vi "Main.Launcher.vi"() -> ()   [LabVIEW 2024]
uses:
  comic_manager/manager_daemon/manager_daemon.lvclass/manager_daemon.ctl
  comic_manager/manager_daemon/manager_daemon.lvclass
  <vilib>/addons/_JKI Toolkits/State Machine/_JKI_lib_State_Machine.llb/Select State(s)_err__jki_lib_state_machine.vi
  <vilib>/addons/_JKI Toolkits/State Machine/_JKI_lib_State_Machine.llb/Periodic Trigger__ogtk__JKI-SM__jki_lib_state_machine.vi
panel:
  out "manager running":bool
  in  "save indices":bool
  in  "launch crawler":bool
  in  "launch interface":bool
  in  "launch graphic UI":bool
  in  "generate indices":bool
  in  "Exit":bool
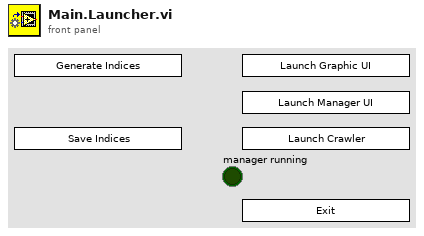
[diagram p1: front panel]
types:
  T1 = enum32{"Invalid", "Standard", "Closed", "Hidden", "Minimized", "Maximized"}
  T2 = enum32{"invalid app kind", "Development System", "Run Time System", "Student Edition", "Embedded LabVIEW", "Evaluation", "Custom"}
  T3 = cluster{"Core":cluster{"Current VI Reference":refnum<vi>, "Close Panel on Exit?":bool}, "manager_daemon":refnum<class "manager_daemon.lvclass">}
  T4 = cluster{"Current VI Reference":refnum<vi>, "Close Panel on Exit?":bool}
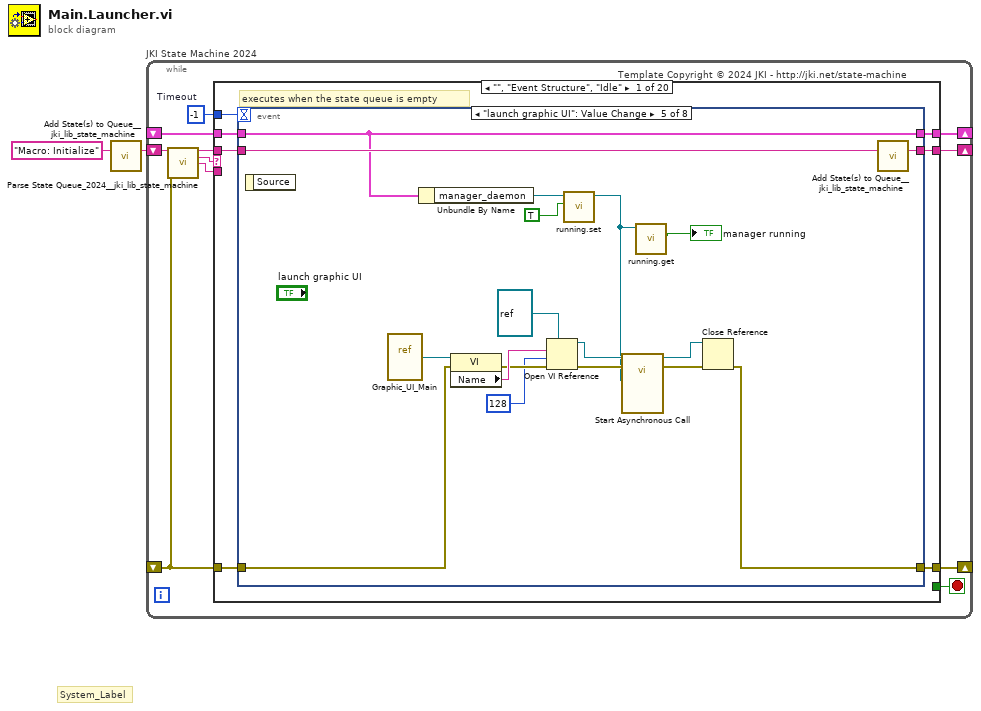
[diagram p0: block diagram]
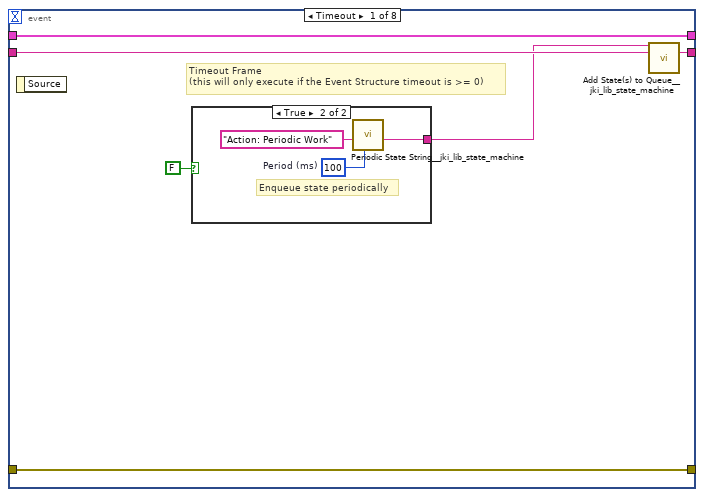
[diagram p2: hidden frame]
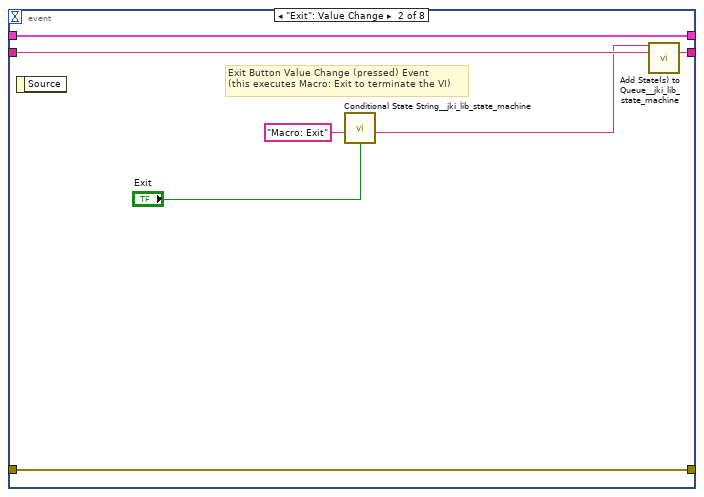
[diagram p4: hidden frame]
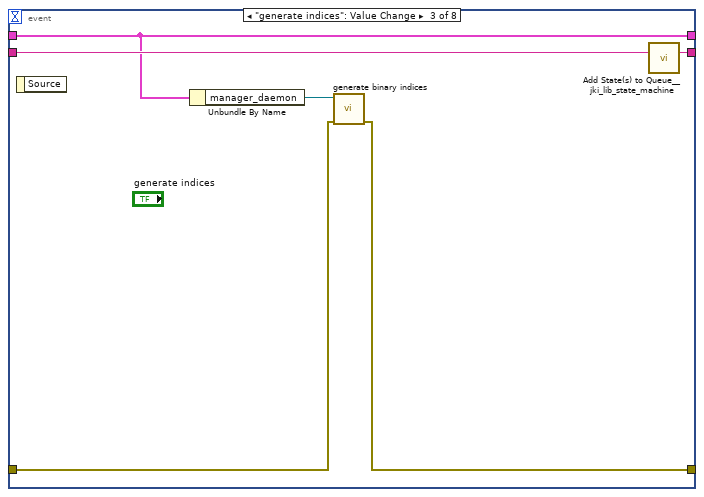
[diagram p5: hidden frame]
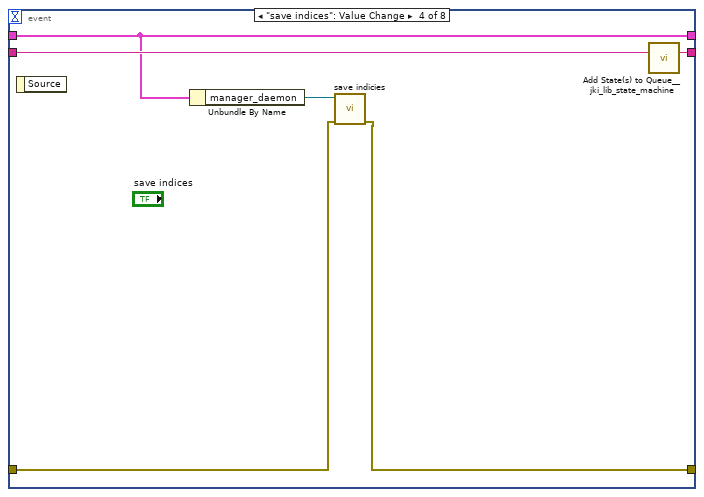
[diagram p6: hidden frame]
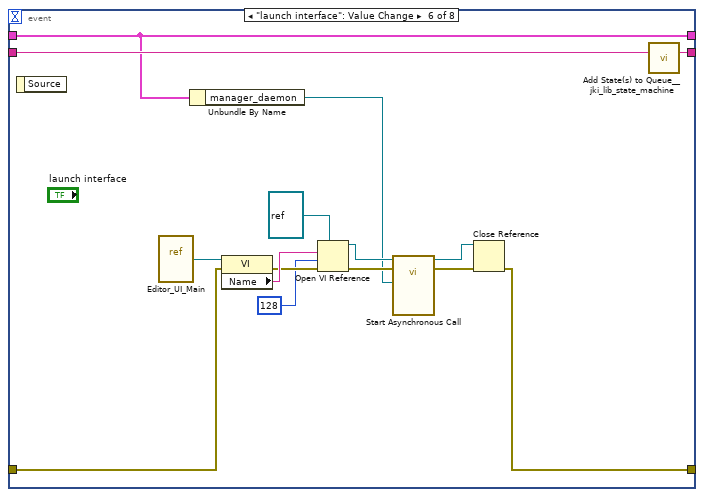
[diagram p7: hidden frame]
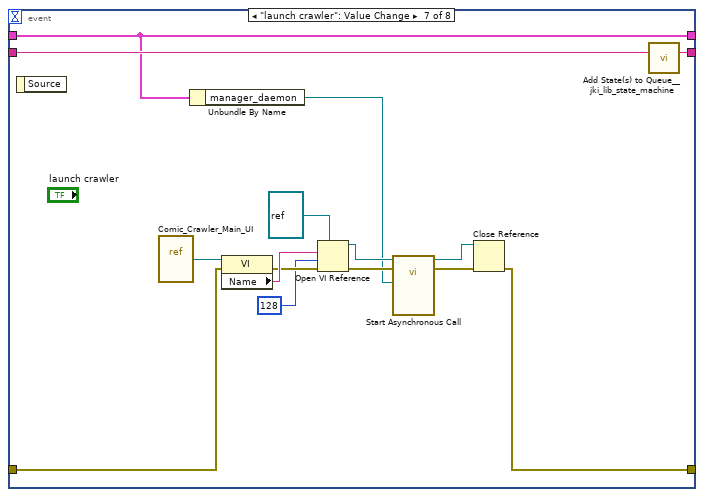
[diagram p8: hidden frame]
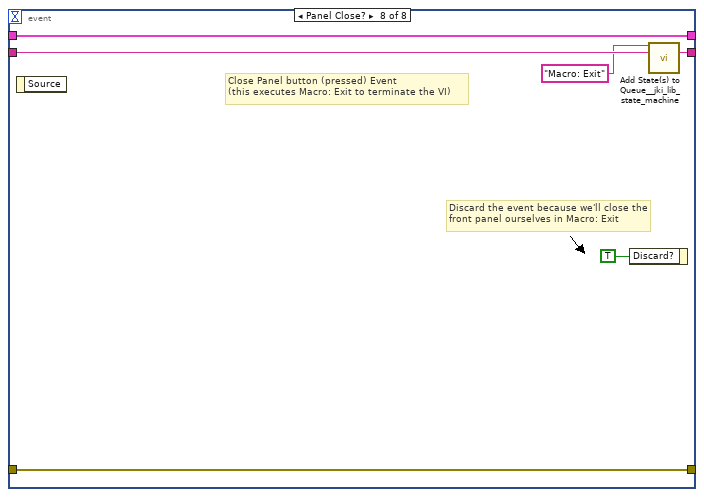
[diagram p9: hidden frame]
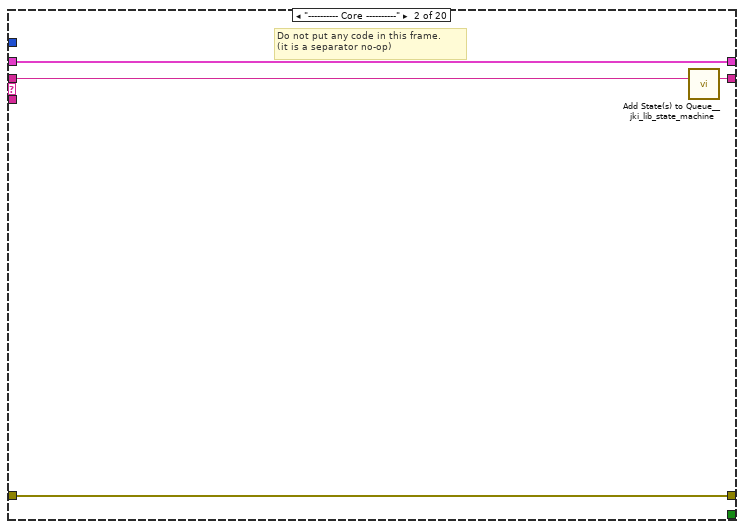
[diagram p10: hidden frame]
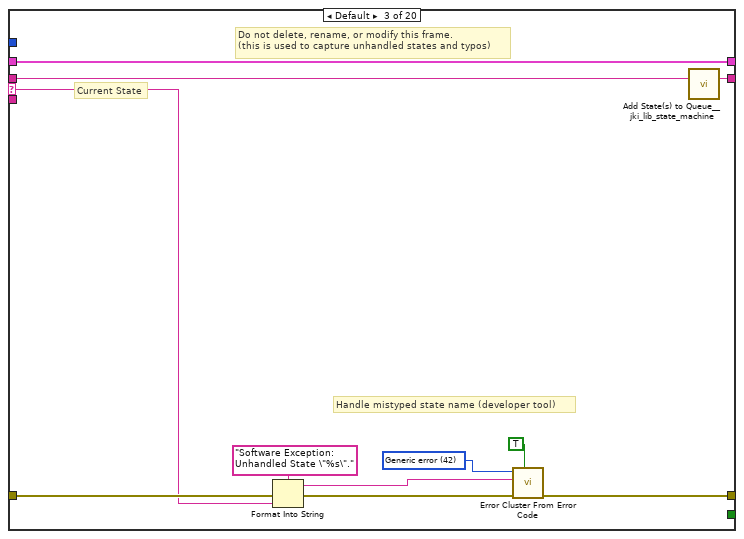
[diagram p11: hidden frame]
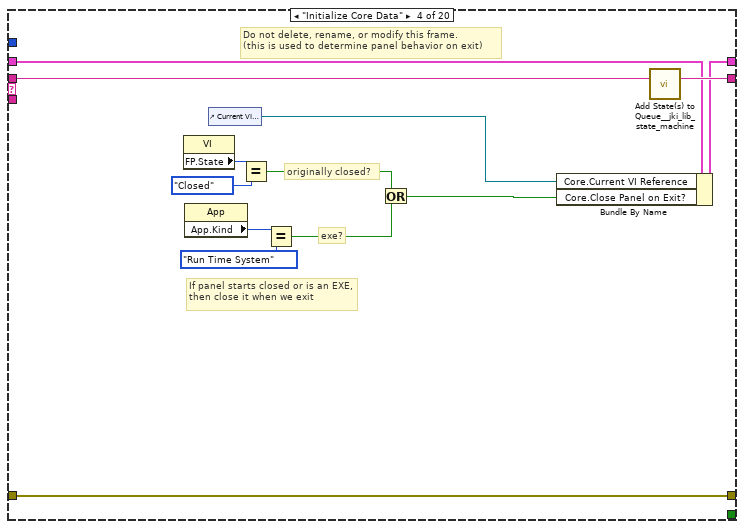
[diagram p12: hidden frame]
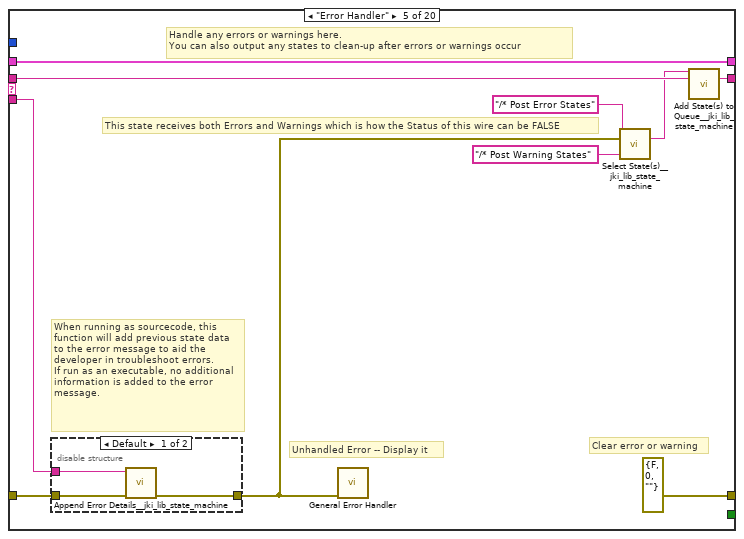
[diagram p13: hidden frame]
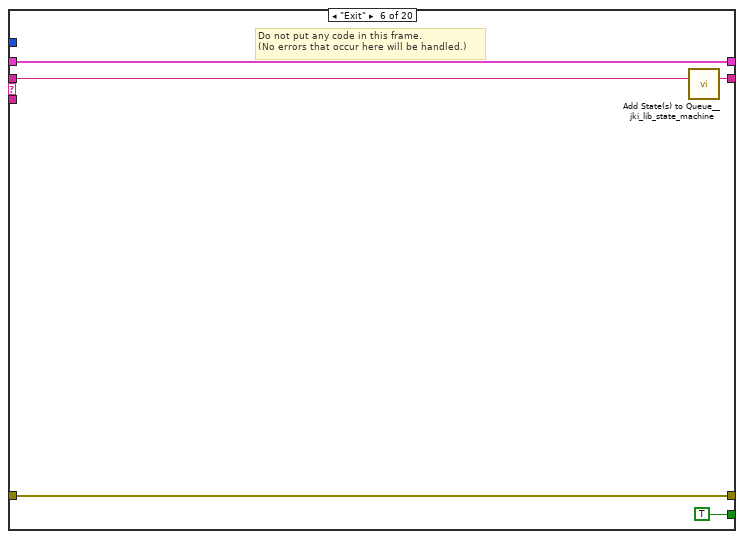
[diagram p15: hidden frame]
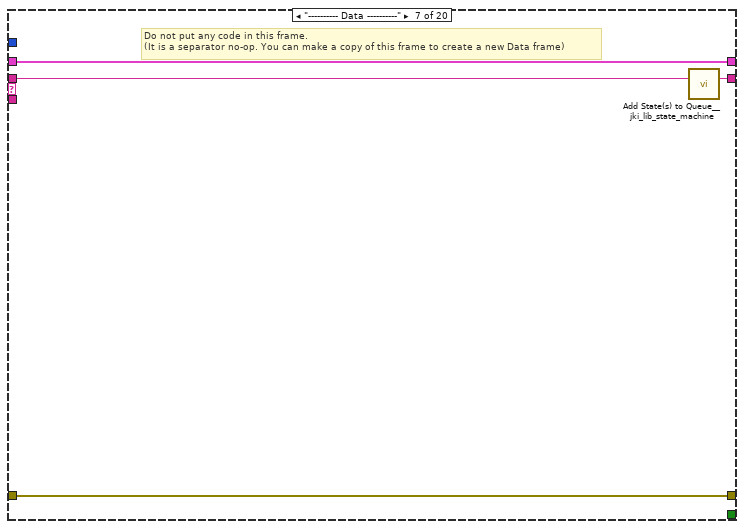
[diagram p16: hidden frame]
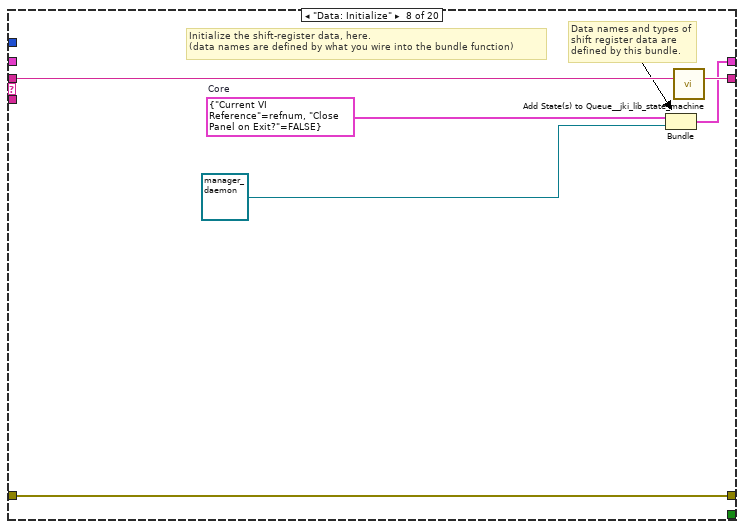
[diagram p17: hidden frame]
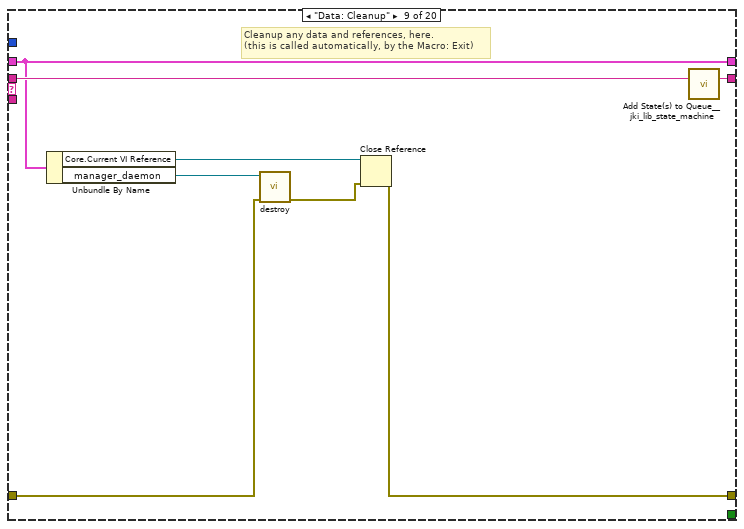
[diagram p18: hidden frame]
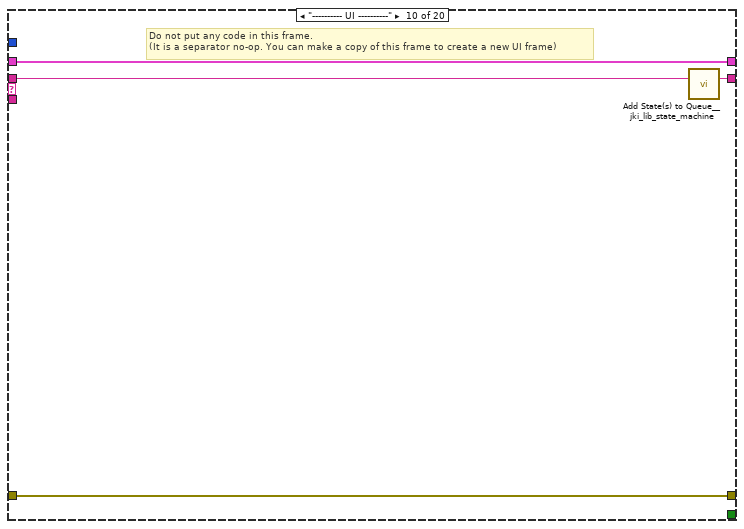
[diagram p19: hidden frame]
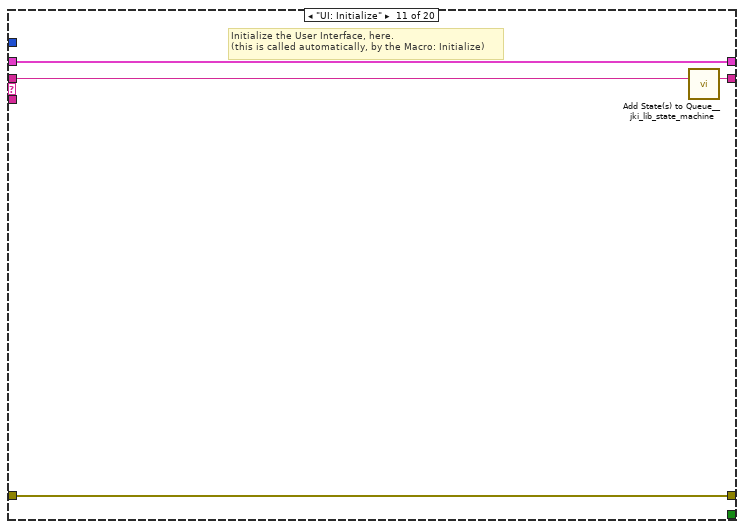
[diagram p20: hidden frame]
diagram:
  # "System_Label"
  n1 = call <vilib>:"Add State(s) to Queue__jki_lib_state_machine.vi"("State(s) in (\"\")"="Macro: Initialize") -> ("States Out"=w2:string)  [unwired: 14 in]
  n2 = while "JKI State Machine 2024" {
    shift-right: [w6] -> _
    shift-left: _ -> [w5]
    shift-right: [w9] -> _
    shift-left: _ -> [w3]
    shift-right: [w8] -> _
    shift-left: w2 -> [w10]
    stop <- w7 stop-if-true
    w4 = -1  # Timeout
    # "Template Copyright © 2024 JKI - http://jki.net/state-machine"
    n3 = call <vilib>:"Parse State Queue_2024__jki_lib_state_machine.vi"("State Queue"=w10, "Error In (no error)"=w3) -> ("Remaining States"=w12:string, "Current State"=w13:string, "Arguments"=w11:string)  [unwired: 11 in]
    n4 = case shown="\"\", \"Event Structure\", \"Idle\"" w13 {
      selector: w13 -> [_ _ w107 _ _ _ _ _ _ _ _ _ _ _ _ _ _ _ _ _]
      tunnel: w12 -> [w20 w106 w111 w130 w140 w149 w153 w159 w167 w171 w175 w179 w185 w196 w265 w270 w279 w283 w289 w300]
      tunnel: w11 -> [_ _ _ _ w135 _ _ _ _ _ _ _ w180 w190 _ _ _ _ _ _]
      tunnel: w5 -> [w18 w103 w109 w123 w137 w147 w150 _ w163 w168 w173 w177 w183 w192 w262 w267 w277 w280 w287 w292]
      tunnel: [w17 w104 w113 w127 errorcluster {"status"=FALSE, "code"=0, "source"=""} ("error out") w145 w151 w156 w164 w169 w172 w176 w181 w193 w263 w268 w271 w281 w284 w294] -> w9
      tunnel: w3 -> [w14 w104 w112 w127 w136 w145 w151 w156 w160 w169 w172 w176 w182 w194 w263 w268 w271 w281 w285 w293]
      tunnel: [w19 w105 w110 w129 w139 w148 w152 w158 w166 w170 w174 w178 w184 w195 w264 w269 w278 w282 w288 w299] -> w8
      tunnel: [_ _ _ _ _ TRUE _ _ _ _ _ _ _ _ _ _ _ _ _ _] -> w7
      tunnel: [w16 w103 w109 w128 w137 w147 w150 w157 w163 w168 w173 w177 w183 w192 w262 w267 w277 w280 w287 w290] -> w6
      tunnel: w4 -> [w15 _ _ _ _ _ _ _ _ _ _ _ _ _ _ _ _ _ _ _]
      frame "", "Event Structure", "Idle" {
        # "executes when the state queue is empty"
        n5 = event shown="[4] \"launch graphic UI\": Value Change" {
          selector: _ -> [_ _ _ _ _ _ _ _]
          dyn-events: _ -> [_ _ _ _ _ _ _ _]
          timeout: w15 -> [_ _ _ _ _ _ _ _]
          tunnel: w20 -> [w26 w36 w42 w48 w66 w81 w96 w102]
          tunnel: [w25 w35 w41 w47 w65 w80 w95 w101] -> w19
          tunnel: w18 -> [w23 w33 w40 w46 w64 w79 w94 w99]
          tunnel: [w24 w34 w37 w43 w53 w67 w82 w100] -> w17
          tunnel: w14 -> [w24 w34 w38 w44 w54 w69 w84 w100]
          tunnel: [w23 w33 w40 w46 w64 w79 w94 w99] -> w16
          event Timeout {
            # "Timeout Frame\n(this will only execute if the Event Structure timeout is >= 0)"
            n6 = event-data() -> ()  [unwired: 1 in, 1 out]
            n7 = case shown="True" FALSE {
              tunnel: [_ w29] -> w22
              frame False {
              }
              frame True {
                w27 = u32 100  # Period (ms)
                # "Enqueue state periodically"
                n8 = call <vilib>:"Periodic State String__jki_lib_state_machine.vi"("Period (ms)"=w27, "State"="Action: Periodic Work") -> ("State Out"=w29:string)  [unwired: 9 in]
              }
            }
            n9 = call <vilib>:"Add State(s) to Queue__jki_lib_state_machine.vi"("State(s) in Front (\"\")"=w22, "State(s) in (\"\")"=w26) -> ("States Out"=w25:string)  [unwired: 13 in]
          }
          event "Exit": Value Change {
            # "Exit Button Value Change (pressed) Event\n(this executes Macro: Exit to terminate the VI)"
            n10 = event-data() -> ()  [unwired: 1 in, 1 out]
            n11 = call <vilib>:"Conditional State String__jki_lib_state_machine.vi"("Do State(s)?"="Exit", "State"="Macro: Exit") -> ("State Out"=w30:string)  [unwired: 7 in]
            n12 = call <vilib>:"Add State(s) to Queue__jki_lib_state_machine.vi"("State(s) in Front (\"\")"=w30, "State(s) in (\"\")"=w36) -> ("States Out"=w35:string)  [unwired: 13 in]
          }
          event "generate indices": Value Change {
            n13 = event-data() -> ()  [unwired: 1 in, 1 out]
            n14 = Unbundle By Name(w40) -> ("manager_daemon"=w39:refnum<class "manager_daemon.lvclass">)
            n15 = call "generate binary indices.vi"("error in (no error)"=w38, "manager_daemon in"=w39) -> ("error out"=w37:errorcluster)  [unwired: 8 in, 1 out]
            n16 = call <vilib>:"Add State(s) to Queue__jki_lib_state_machine.vi"("State(s) in (\"\")"=w42) -> ("States Out"=w41:string)  [unwired: 14 in]
          }
          event "save indices": Value Change {
            n17 = event-data() -> ()  [unwired: 1 in, 1 out]
            n18 = Unbundle By Name(w46) -> ("manager_daemon"=w45:refnum<class "manager_daemon.lvclass">)
            n19 = call "save indicies.vi"("error in (no error)"=w44, "manager_daemon in"=w45) -> ("error out"=w43:errorcluster)  [unwired: 8 in, 1 out]
            n20 = call <vilib>:"Add State(s) to Queue__jki_lib_state_machine.vi"("State(s) in (\"\")"=w48) -> ("States Out"=w47:string)  [unwired: 14 in]
          }
          event "launch graphic UI": Value Change {
            n21 = event-data() -> ()  [unwired: 1 in, 1 out]
            n22 = vi-ref "Graphic_UI_Main.vi"() -> (w56:refnum<vi>)
            n23 = Unbundle By Name(w64) -> ("manager_daemon"=w51:refnum<class "manager_daemon.lvclass">)
            n24 = property class="VI"(reference=w56, error in=w54) -> (error out=w57:errorcluster, "Name"=w58:string)  [unwired: 1 out]
            n25 = Open VI Reference(type specifier VI Refnum (for type only)=refnum<vi> refnum, vi path=w58, options=128, error in (no error)=w57) -> (vi reference=w60:refnum<vi>, error out=w63:errorcluster)  [unwired: 2 in]
            n26 = call "running.set.vi"("running"=TRUE, "manager_daemon in"=w51) -> ("manager_daemon out"=w50:refnum<class "manager_daemon.lvclass">)  [unwired: 9 in]
            n27 = call-by-ref "Start Asynchronous Call"(reference=w60, error in=w63, "manager_daemon"=w50) -> (reference out=w61:refnum<vi>, error out=w62:errorcluster)  [unwired: 11 in]
            n28 = call "running.get.vi"("manager_daemon in"=w50) -> ("manager running"=→"manager running":bool)  [unwired: 9 in, 1 out]
            n29 = Close Reference(reference=w61, error in (no error)=w62) -> (error out=w53:errorcluster)
            n30 = call <vilib>:"Add State(s) to Queue__jki_lib_state_machine.vi"("State(s) in (\"\")"=w66) -> ("States Out"=w65:string)  [unwired: 14 in]
          }
          event "launch interface": Value Change {
            n31 = event-data() -> ()  [unwired: 1 in, 1 out]
            n32 = vi-ref "Editor_UI_Main.vi"() -> (w71:refnum<vi>)
            n33 = Unbundle By Name(w79) -> ("manager_daemon"=w68:refnum<class "manager_daemon.lvclass">)
            n34 = property class="VI"(reference=w71, error in=w69) -> (error out=w72:errorcluster, "Name"=w73:string)  [unwired: 1 out]
            n35 = Open VI Reference(type specifier VI Refnum (for type only)=refnum<vi> refnum, vi path=w73, options=128, error in (no error)=w72) -> (vi reference=w75:refnum<vi>, error out=w78:errorcluster)  [unwired: 2 in]
            n36 = call-by-ref "Start Asynchronous Call"(reference=w75, error in=w78, "manager_daemon"=w68) -> (reference out=w76:refnum<vi>, error out=w77:errorcluster)  [unwired: 11 in]
            n37 = Close Reference(reference=w76, error in (no error)=w77) -> (error out=w67:errorcluster)
            n38 = call <vilib>:"Add State(s) to Queue__jki_lib_state_machine.vi"("State(s) in (\"\")"=w81) -> ("States Out"=w80:string)  [unwired: 14 in]
          }
          event "launch crawler": Value Change {
            n39 = event-data() -> ()  [unwired: 1 in, 1 out]
            n40 = vi-ref "Comic_Crawler_Main_UI.vi"() -> (w86:refnum<vi>)
            n41 = Unbundle By Name(w94) -> ("manager_daemon"=w83:refnum<class "manager_daemon.lvclass">)
            n42 = property class="VI"(reference=w86, error in=w84) -> (error out=w87:errorcluster, "Name"=w88:string)  [unwired: 1 out]
            n43 = Open VI Reference(type specifier VI Refnum (for type only)=refnum<vi> refnum, vi path=w88, options=128, error in (no error)=w87) -> (vi reference=w90:refnum<vi>, error out=w93:errorcluster)  [unwired: 2 in]
            n44 = call-by-ref "Start Asynchronous Call"(reference=w90, error in=w93, "manager_daemon"=w83) -> (reference out=w91:refnum<vi>, error out=w92:errorcluster)  [unwired: 11 in]
            n45 = Close Reference(reference=w91, error in (no error)=w92) -> (error out=w82:errorcluster)
            n46 = call <vilib>:"Add State(s) to Queue__jki_lib_state_machine.vi"("State(s) in (\"\")"=w96) -> ("States Out"=w95:string)  [unwired: 14 in]
          }
          event Panel Close? {
            # "Discard the event because we'll close the front panel ourselves in Macro: Exit"
            # "Close Panel button (pressed) Event\n(this executes Macro: Exit to terminate the VI)"
            n47 = event-data() -> ()  [unwired: 1 in, 1 out]
            n48 = event-data("Discard?"=TRUE) -> ()  [unwired: 1 in, 1 out]
            n49 = call <vilib>:"Add State(s) to Queue__jki_lib_state_machine.vi"("State(s) in Front (\"\")"="Macro: Exit", "State(s) in (\"\")"=w102) -> ("States Out"=w101:string)  [unwired: 13 in]
          }
        }
      }
      frame "---------- Core ----------" {
        # "Do not put any code in this frame.\n(it is a separator no-op)"
        n50 = call <vilib>:"Add State(s) to Queue__jki_lib_state_machine.vi"("State(s) in (\"\")"=w106) -> ("States Out"=w105:string)  [unwired: 14 in]
      }
      frame Default {
        w116 = 42 items=["No error", "Argument error", "Memory is full", "Out of zone", "End of file", "File already open", "Generic file I/O error", "File not found", "File permission error", "Disk is full", "Duplicate path", "Too many files open", "System feature not enabled", "Resource file not found", "Cannot add resource", "Resource not found", "Image not found", "Image memory error", "Pen does not exist", "Config type invalid", "Config token not found", "Config parse error", "Config memory error", "Bad external code format", "Bad external code offset", "External code not present", "Null window", "Destroy window error", "Null menu", "Print aborted", "Bad print record", "Print driver error", "Windows error during printing", "Memory error during printing", "Print dialog error", "Generic print error", "Invalid device refnum", "Device not found", "Device parameter error", "Device unit error", "Cannot open device", "Device call aborted", "Generic error", "Cancelled by user", "Object ID too low", "Object ID too high", "Object not in heap", "Unknown heap", "Unknown object (invalid DefProc)", "Unknown object (DefProc not in table)", "Message out of range", "Invalid (null) method", "Unknown message", "Manager call not supported", "Bad address", "Network operation in progress", "Network operation timed out", "Connection is busy", "Network attribute not supported", "Network error", "Address in use", "System out of memory", "Connection aborted", "Connection refused", "Not connected", "Already connected", "Connection closed", "Initialization error (interapplication manager)", "Bad occurrence", "Wait on unbound occurrence handler", "Occurrence queue overflow", "Datalog type conflict", "Unused", "Unrecognized type (interapplication manager)", "Memory corrupt", "Failed to make temporary DLL", "Old CIN version", "Drag socket not found", "Failed to load drop-object", "Failed to register OLE object", "Failed to release OLE object", "Format specifier type mismatch", "Unknown format specifier", "Too few format specifiers", "Too many format specifiers", "Scan failed", "Newer CIN version", "Error converting to variant", "Runtime menu error", "Password tampered", "Variant attribute not found", "Incompatible variant data type", "Event data is not available", "Event Store is not present", "Occurrence is not found", "Event Queue is not created", "Event info is not available", "Refnum passed is NULL", "Error retrieving Class GUID", "Error retrieving CoClass GUID", "Error retrieving TypeLib GUID.", "Bad built application magic bytes.", "Specific driver is different from the specific driver associated with the Logical Name.", "There is no session opened to the class driver.", "Max Error", "MAX - Error with config objects", "MAX - Error loading configuration", "MAX - Group not supported"]
        # "Current State"
        # "Do not delete, rename, or modify this frame.\n(this is used to capture unhandled states and typos)"
        # "Handle mistyped state name (developer tool)"
        n51 = Format Into String(format string="Software Exception: Unhandled State \"%s\"." ("message"), error in=w112, w107) -> (resulting string=w115:string, error out=w114:errorcluster)  [unwired: 1 in]
        n52 = call <vilib>:"Error Cluster From Error Code.vi"("show call chain? (False)"=TRUE, "error in (no error)"=w114, "error message (\"\")"=w115, "error code (0)"=w116) -> ("error out"=w113:errorcluster)  [unwired: 5 in]
        n53 = call <vilib>:"Add State(s) to Queue__jki_lib_state_machine.vi"("State(s) in (\"\")"=w111) -> ("States Out"=w110:string)  [unwired: 14 in]
      }
      frame "Initialize Core Data" {
        # "Do not delete, rename, or modify this frame.\n(this is used to determine panel behavior on exit)"
        # "originally closed?"
        # "exe?"
        # "If panel starts closed or is an EXE, then close it when we exit"
        n54 = property class="VI"() -> ("FP.State"=w120:T1)  [unwired: 2 in, 2 out]
        n55 = property class="App"() -> ("App.Kind"=w126:T2)  [unwired: 2 in, 2 out]
        n56 = control-ref of="Current VI Reference"() -> (w121:refnum<vi>)
        n57 = Equal?(x=w120, y=T1."Closed" ("Front Panel Window:State")) -> (x = y?=w118:bool)
        n58 = Equal?(x=w126, y=T2."Run Time System" ("Application:Kind")) -> (x = y?=w124:bool)
        n59 = Or(x=w118, y=w124) -> (x .or. y?=w122:bool)
        n60 = Bundle By Name(cluster=w123, "Core.Current VI Reference"=w121, "Core.Close Panel on Exit?"=w122) -> (w128:T3)
        n61 = call <vilib>:"Add State(s) to Queue__jki_lib_state_machine.vi"("State(s) in (\"\")"=w130) -> ("States Out"=w129:string)  [unwired: 14 in]
      }
      frame "Error Handler" {
        # "When running as sourcecode, this function will add previous state data to the error message to aid the developer in troubleshoot errors.\nIf run as an executable, no additional information is added to the error message."
        # "This state receives both Errors and Warnings which is how the Status of this wire can be FALSE"
        # "Unhandled Error -- Display it"
        # "Handle any errors or warnings here.\nYou can also output any states to clean-up after errors or warnings occur"
        # "Clear error or warning"
        n62 = disable-structure shown="Default" {
          disable-tunnel: w136 -> [w143 w144]
          disable-tunnel: w135 -> [w142 _]
          disable-tunnel: [w141 w144] -> w134
          frame condition #0 (active) {
            n63 = call <vilib>:"Append Error Details__jki_lib_state_machine.vi"("error in (no error)"=w143, "Previous State and Argument(s)"=w142) -> ("error out"=w141:errorcluster)  [unwired: 9 in]
          }
          frame condition #1 {
          }
        }
        n64 = call <vilib>:"General Error Handler.vi"("error in (no error)"=w134) -> ()  [unwired: 10 in, 5 out]
        n65 = call-poly <vilib>:"Select State(s)__jki_lib_state_machine.vi"("State(s) if True (\"\")"="/* Post Error States", "Select"=w134, "State(s) if False (\"\")"="/* Post Warning States") -> ("States Out"=w132:string)  [unwired: 12 in]
        n66 = call <vilib>:"Add State(s) to Queue__jki_lib_state_machine.vi"("State(s) in Front (\"\")"=w132, "State(s) in (\"\")"=w140) -> ("States Out"=w139:string)  [unwired: 13 in]
      }
      frame "Exit" {
        # "Do not put any code in this frame.\n(No errors that occur here will be handled.)"
        n67 = call <vilib>:"Add State(s) to Queue__jki_lib_state_machine.vi"("State(s) in (\"\")"=w149) -> ("States Out"=w148:string)  [unwired: 14 in]
      }
      frame "---------- Data ----------" {
        # "Do not put any code in this frame.\n(It is a separator no-op. You can make a copy of this frame to create a new Data frame)"
        n68 = call <vilib>:"Add State(s) to Queue__jki_lib_state_machine.vi"("State(s) in (\"\")"=w153) -> ("States Out"=w152:string)  [unwired: 14 in]
      }
      frame "Data: Initialize" {
        w155 = T4 {"Current VI Reference"=refnum, "Close Panel on Exit?"=FALSE}  # Core
        # "Data names and types of shift register data are defined by this bundle."
        # "Initialize the shift-register data, here.\n(data names are defined by what you wire into the bundle function)"
        n69 = Bundle("Core"=w155, "manager_daemon"=refnum<class "manager_daemon.lvclass"> refnum) -> (w157:T3)  [unwired: 1 in]
        n70 = call <vilib>:"Add State(s) to Queue__jki_lib_state_machine.vi"("State(s) in (\"\")"=w159) -> ("States Out"=w158:string)  [unwired: 14 in]
      }
      frame "Data: Cleanup" {
        # "Cleanup any data and references, here.\n(this is called automatically, by the Macro: Exit)"
        n71 = Unbundle By Name(w163) -> ("Core.Current VI Reference"=w165:refnum<vi>, "manager_daemon"=w162:refnum<class "manager_daemon.lvclass">)
        n72 = call "destroy.vi"("error in (no error)"=w160, "manager_daemon in"=w162) -> ("error out"=w161:errorcluster)  [unwired: 8 in, 1 out]
        n73 = Close Reference(reference=w165, error in (no error)=w161) -> (error out=w164:errorcluster)
        n74 = call <vilib>:"Add State(s) to Queue__jki_lib_state_machine.vi"("State(s) in (\"\")"=w167) -> ("States Out"=w166:string)  [unwired: 14 in]
      }
      frame "---------- UI ----------" {
        # "Do not put any code in this frame.\n(It is a separator no-op. You can make a copy of this frame to create a new UI frame)"
        n75 = call <vilib>:"Add State(s) to Queue__jki_lib_state_machine.vi"("State(s) in (\"\")"=w171) -> ("States Out"=w170:string)  [unwired: 14 in]
      }
      frame "UI: Initialize" {
        # "Initialize the User Interface, here.\n(this is called automatically, by the Macro: Initialize)"
        n76 = call <vilib>:"Add State(s) to Queue__jki_lib_state_machine.vi"("State(s) in (\"\")"=w175) -> ("States Out"=w174:string)  [unwired: 14 in]
      }
      frame "UI: Uninitialize" {
        # "Cleanup the User Interface, here.\n(this is called automatically, by the Macro: Exit)"
        n77 = call <vilib>:"Add State(s) to Queue__jki_lib_state_machine.vi"("State(s) in (\"\")"=w179) -> ("States Out"=w178:string)  [unwired: 14 in]
      }
      frame "UI: Cursor Set" {
        # "Argument"
        # "Set and Unset Cursor Busy.\n(Usage: \"UI: Cursor Set >> Busy|Idle\")"
        n78 = case shown="\"Idle\", Default" w180 {
          tunnel: w182 -> [w187 w189]
          tunnel: [w186 w188] -> w181
          frame "Idle", Default {
            n79 = call <vilib>:"Unset Busy.vi"("error in (no error)"=w187) -> ("error out"=w186:errorcluster)  [unwired: 10 in]
          }
          frame "Busy" {
            n80 = call <vilib>:"Set Busy.vi"("error in (no error)"=w189) -> ("error out"=w188:errorcluster)  [unwired: 9 in, 1 out]
          }
        }
        n81 = call <vilib>:"Add State(s) to Queue__jki_lib_state_machine.vi"("State(s) in (\"\")"=w185) -> ("States Out"=w184:string)  [unwired: 14 in]
      }
      frame "UI: Front Panel State" {
        # "Argument"
        # "Set Front Panel Open or Closed\n(Usage: \"UI: Front Panel State >> Open|Close\")"
        n82 = Unbundle By Name(w192) -> ("Core.Current VI Reference"=w191:refnum<vi>)
        n83 = case shown="\"Minimize\", \"Minimized\"" w190 {
          tunnel: w194 -> [w202 w217 w228 w241 w254]
          tunnel: [w204 w218 w230 w243 w256] -> w193
          tunnel: w191 -> [w203 w215 w229 w242 w255]
          frame "Open", "Standard", Default {
            w197 = T1."Standard" ("State")
            n84 = property class="VI"(reference=w203, error in=w202) -> (reference out=w200:refnum<vi>, error out=w201:errorcluster, "FP.State"=w199:T1)
            n85 = Not Equal?(x=w199, y=w197) -> (x != y?=w198:bool)
            n86 = case shown="True" w198 {
              tunnel: [w208 w210] -> w204
              tunnel: w201 -> [w207 w210]
              tunnel: w200 -> [w206 _]
              tunnel: w197 -> [w205 _]
              frame True {
                n87 = invoke class="VI" method="FP.Open"(reference=w206, error in=w207, "Activate"=TRUE, "State"=w205) -> (error out=w208:errorcluster)  [unwired: 1 in, 4 out]
              }
              frame False {
              }
            }
          }
          frame "Close", "Closed" {
            n88 = property class="VI"(reference=w215, error in=w217) -> (reference out=w214:refnum<vi>, error out=w216:errorcluster, "FP.State"=w212:T1)
            n89 = Not Equal?(x=w212, y=T1."Closed" ("Front Panel Window:State")) -> (x != y?=w211:bool)
            n90 = case shown="True" w211 {
              tunnel: [w219 w222] -> w218
              tunnel: w216 -> [w219 w221]
              tunnel: w214 -> [_ w220]
              frame False {
              }
              frame True {
                n91 = invoke class="VI" method="FP.Close"(reference=w220, error in=w221) -> (error out=w222:errorcluster)  [unwired: 1 in, 2 out]
              }
            }
          }
          frame "Hidden", "Hide" {
            w223 = T1."Hidden" ("State")
            n92 = property class="VI"(reference=w229, error in=w228) -> (reference out=w226:refnum<vi>, error out=w227:errorcluster, "FP.State"=w225:T1)
            n93 = Not Equal?(x=w225, y=w223) -> (x != y?=w224:bool)
            n94 = case shown="True" w224 {
              tunnel: [w234 w235] -> w230
              tunnel: w227 -> [w233 w235]
              tunnel: w226 -> [w232 _]
              tunnel: w223 -> [w231 _]
              frame True {
                n95 = invoke class="VI" method="FP.Open"(reference=w232, error in=w233, "State"=w231) -> (error out=w234:errorcluster)  [unwired: 2 in, 4 out]
              }
              frame False {
              }
            }
          }
          frame "Minimize", "Minimized" {
            w236 = T1."Minimized" ("State")
            n96 = property class="VI"(reference=w242, error in=w241) -> (reference out=w239:refnum<vi>, error out=w240:errorcluster, "FP.State"=w238:T1)
            n97 = Not Equal?(x=w238, y=w236) -> (x != y?=w237:bool)
            n98 = case shown="True" w237 {
              tunnel: [w247 w248] -> w243
              tunnel: w240 -> [w246 w248]
              tunnel: w239 -> [w245 _]
              tunnel: w236 -> [w244 _]
              frame True {
                n99 = invoke class="VI" method="FP.Open"(reference=w245, error in=w246, "State"=w244) -> (error out=w247:errorcluster)  [unwired: 2 in, 4 out]
              }
              frame False {
              }
            }
          }
          frame "Maximize", "Maximized" {
            w249 = T1."Maximized" ("State")
            n100 = property class="VI"(reference=w255, error in=w254) -> (reference out=w252:refnum<vi>, error out=w253:errorcluster, "FP.State"=w251:T1)
            n101 = Not Equal?(x=w251, y=w249) -> (x != y?=w250:bool)
            n102 = case shown="True" w250 {
              tunnel: [w260 w261] -> w256
              tunnel: w253 -> [w259 w261]
              tunnel: w252 -> [w258 _]
              tunnel: w249 -> [w257 _]
              frame True {
                n103 = invoke class="VI" method="FP.Open"(reference=w258, error in=w259, "State"=w257) -> (error out=w260:errorcluster)  [unwired: 2 in, 4 out]
              }
              frame False {
              }
            }
          }
        }
        n104 = call <vilib>:"Add State(s) to Queue__jki_lib_state_machine.vi"("State(s) in (\"\")"=w196) -> ("States Out"=w195:string)  [unwired: 14 in]
      }
      frame "---------- Macro ----------" {
        # "Do not put any code in this frame.\n(It is a separator no-op. You can make a copy of this frame to create a new Macro frame)"
        n105 = call <vilib>:"Add State(s) to Queue__jki_lib_state_machine.vi"("State(s) in (\"\")"=w265) -> ("States Out"=w264:string)  [unwired: 14 in]
      }
      frame "Macro: Initialize" {
        w266 = "Data: Initialize\nInitialize Core Data\nUI: Initialize\nUI: Front Panel State >> Open\nActions: Start Manager"  # Data: Initialize Initialize Core Data UI: Initialize UI: Front Panel State >> Open Actions: Start Manager
        # "Initialization Macro\n(This is called once, when the VI starts)"
        n106 = call <vilib>:"Add State(s) to Queue__jki_lib_state_machine.vi"("State(s) in Front (\"\")"=w266, "State(s) in (\"\")"=w270) -> ("States Out"=w269:string)  [unwired: 13 in]
      }
      frame "Macro: Exit" {
        # "Exit Macro\n(This is called once, when the VI exits)"
        n107 = Unbundle By Name(w277) -> ("Core.Close Panel on Exit?"=w273:bool)
        n108 = call <vilib>:"Conditional State String__jki_lib_state_machine.vi"("Do State(s)?"=w273, "State"="UI: Front Panel State >> Close") -> ("State Out"=w272:string)  [unwired: 7 in]
        n109 = call <vilib>:"Add State(s) to Queue__jki_lib_state_machine.vi"("State(s) in (\"\")"=w272, "State(s) at Back (\"\")"="Actions: Save Indices\nUI: Uninitialize\nData: Cleanup\nExit") -> ("States Out"=w275:string)  [unwired: 13 in]
        n110 = call <vilib>:"Add State(s) to Queue__jki_lib_state_machine.vi"("State(s) in Front (\"\")"=w275, "State(s) in (\"\")"=w279) -> ("States Out"=w278:string)  [unwired: 13 in]
      }
      frame "---------- Actions ----------" {
        # "Template Separator\n(You can make a copy of, or modify, this frame)"
        n111 = call <vilib>:"Add State(s) to Queue__jki_lib_state_machine.vi"("State(s) in (\"\")"=w283) -> ("States Out"=w282:string)  [unwired: 14 in]
      }
      frame "Actions: Save Indices" {
        n112 = Unbundle By Name(w287) -> ("manager_daemon"=w286:refnum<class "manager_daemon.lvclass">)
        n113 = call "save indicies.vi"("error in (no error)"=w285, "manager_daemon in"=w286) -> ("error out"=w284:errorcluster)  [unwired: 8 in, 1 out]
        n114 = call <vilib>:"Add State(s) to Queue__jki_lib_state_machine.vi"("State(s) in (\"\")"=w289) -> ("States Out"=w288:string)  [unwired: 14 in]
      }
      frame "Actions: Start Manager" {
        n115 = call "create.vi"("error in (no error)"=w293) -> ("error out"=w296:errorcluster, "manager_daemon out"=w298:refnum<class "manager_daemon.lvclass">)  [unwired: 9 in]
        n116 = call "start.vi"("error in (no error)"=w296, "manager_daemon in"=w298) -> ("error out"=w295:errorcluster, "manager_daemon out"=w297:refnum<class "manager_daemon.lvclass">)  [unwired: 8 in]
        n117 = call "load indices.vi"("error in (no error)"=w295, "manager_daemon in"=w297) -> ("error out"=w294:errorcluster, "manager_daemon out"=w291:refnum<class "manager_daemon.lvclass">)  [unwired: 8 in]
        n118 = Bundle By Name(cluster=w292, "manager_daemon"=w291) -> (w290:T3)
        n119 = call <vilib>:"Add State(s) to Queue__jki_lib_state_machine.vi"("State(s) in (\"\")"=w300) -> ("States Out"=w299:string)  [unwired: 14 in]
      }
    }
  }
